vi "Resize.vi"(9 "Container State":T1, 11 "Display State In":T2) -> ()   [LabVIEW 2019, in "ExpandHorizontal.xctl"]
uses:
  ExpandHorizontal.xctl
  State.ctl
  <vilib>/_xctls/Container State.ctl
  <vilib>/_xctls/XControlSupport.lvlib
panel:
  out "error out":errorcluster
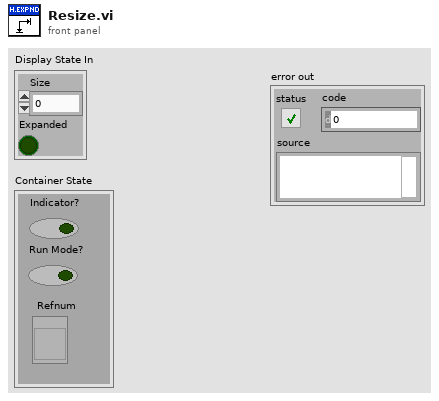
[diagram p1: front panel]
types:
  T1 = typedef "XControlSupport.lvlib/Container State.ctl" = cluster{"Indicator?":bool, "Run Mode?":bool, " Refnum":refnum<vi>}
  T2 = typedef "ExpandHorizontal.xctl/State.ctl" = cluster{"Size":i16, "Expanded":bool}
  T3 = typedef "LVRectTypeDef.ctl" = cluster{"Left":i16, "Top":i16, "Right":i16, "Bottom":i16}
  T4 = typedef "LVPointTypeDef.ctl" = cluster{"Horizontal":i16, "Vertical":i16}
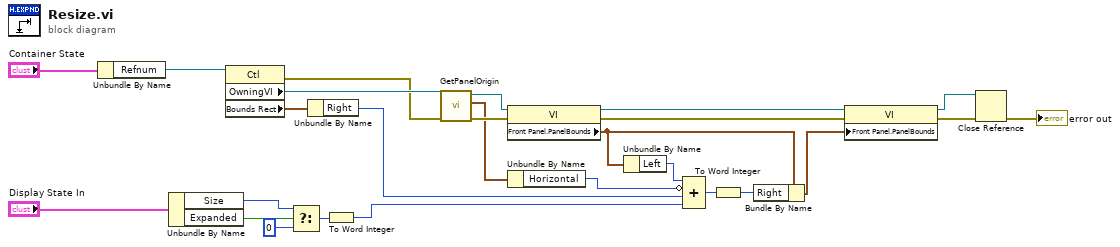
[diagram p0: block diagram]
diagram:
  n1 = Unbundle By Name("Container State") -> ("Refnum"=w24:refnum<vi>)
  n2 = Unbundle By Name("Display State In") -> ("Size"=w21:i16, "Expanded"=w22:bool)
  n3 = property class="Ctl"(reference=w24) -> (error out=w8:errorcluster, "OwningVI"=w9:refnum<vi>, "Bounds Rect"=w4:T3)  [unwired: 1 in, 1 out]
  n4 = Select(t=w21, s=w22, f=i16 0) -> (s? t:f=w20:i16)
  n5 = Unbundle By Name(w4) -> ("Right"=w3:i16)
  n6 = To Word Integer(number=w20) -> (16bit integer=w12:i16)
  n7 = call "GetPanelOrigin.vi"("error in (no error)"=w8, "VI in"=w9) -> ("error out"=w7:errorcluster, "Origin"=w2:T4, "VI out"=w6:refnum<vi>)  [unwired: 7 in]
  n8 = property class="VI"(reference=w6, error in=w7) -> (reference out=w5:refnum<vi>, error out=w15:errorcluster, "Front Panel.PanelBounds"=w11:T3)
  n9 = Unbundle By Name(w2) -> ("Horizontal"=w1:i16)
  n10 = Unbundle By Name(w11) -> ("Left"=w10:i16)
  n11 = Compound Arithmetic op=ADD(w10, invert w1, w3, w12) -> (w26:i16)
  n12 = To Word Integer(number=w26) -> (16bit integer=w13:i16)
  n13 = Bundle By Name(cluster=w11, "Right"=w13) -> (w16:T3)
  n14 = property class="VI"(reference=w5, error in=w15, "Front Panel.PanelBounds"=w16) -> (reference out=w18:refnum<vi>, error out=w17:errorcluster)
  n15 = Close Reference(reference=w18, error in (no error)=w17) -> (error out=→"error out":errorcluster)
